vi "Box ID Check.vi"(8 "error in (no error)":errorcluster, 10 "Box ID":u8, 11 "CAN in":refnum<class "XNET_BS120x.lvclass">) -> (0 "error out":errorcluster, 3 "CAN out":refnum<class "XNET_BS120x.lvclass">)   [LabVIEW 2021, in "BS120x Driver.lvlib" / "XNET_BS120x.lvclass"]
uses:
  XNET_BS120x.lvclass
  XNET_BS120x.lvclass/XNET_BS120x.ctl
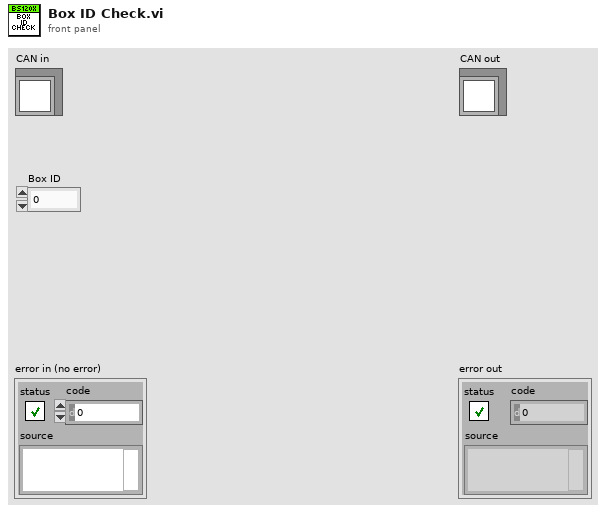
[diagram p1: front panel]
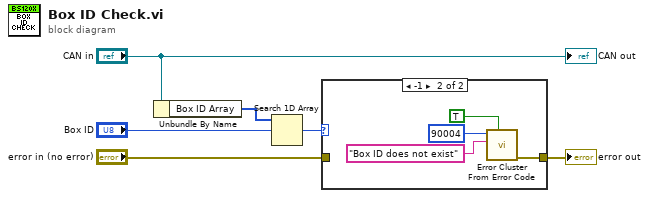
[diagram p0: block diagram]
diagram:
  n1 = Unbundle By Name("CAN in") -> ("Box ID Array"=w2:u8[])
  n2 = Search 1D Array(1D array=w2, element="Box ID") -> (index of element=w1:i32)  [unwired: 1 in]
  n3 = case shown="-1" w1 {
    tunnel: "error in (no error)" -> [w7 _]
    tunnel: [w7 w8] -> w3
    frame Default {
    }
    frame -1 {
      n4 = call <vilib>:"Error Cluster From Error Code.vi"("show call chain? (False)"=TRUE, "error message (\"\")"="Box ID does not exist", "error code (0)"=90004) -> ("error out"=w8:errorcluster)  [unwired: 6 in]
    }
  }
  "error out" <- w3
  "CAN out" <- "CAN in"
